vi "macro_Cmd_FindFollowHolonomicSimpleExecute.vi"() -> ()   [LabVIEW 2019, in "PathPlanner24.lvlib"]
uses:
  <vilib>/Rock Robotics/WPI/ThirdParty/JAS_Junk/TrajLib/TypeDef/CHASSIS_SPEEDS.ctl
  <vilib>/Rock Robotics/WPI/ThirdParty/JAS_Junk/TrajLib/TypeDef/POSE2D.ctl
  <vilib>/Rock Robotics/WPI/ThirdParty/JAS_Junk/TrajLib/TypeDef/TRANSLATION2D.ctl
  <vilib>/Rock Robotics/WPI/ThirdParty/JAS_Junk/TrajLib/TypeDef/ROTATION2D.ctl
  <vilib>/Rock Robotics/WPI/ThirdParty/JAS_Junk/TrajLib/ProfiledPIDController_NewPeriod.vi
  <vilib>/Rock Robotics/WPI/ThirdParty/JAS_Junk/TrajLib/ProfiledPIDController_SetIntegratorRange.vi
  <vilib>/Rock Robotics/WPI/ThirdParty/JAS_Junk/TrajLib/ProfiledPIDController_DisableContInput.vi
  <vilib>/Rock Robotics/WPI/ThirdParty/JAS_Junk/TrajLib/ProfiledPIDController_EnableContInput.vi
  <vilib>/Rock Robotics/WPI/ThirdParty/JAS_Junk/TrajLib/TrapProfConstraint_New.vi
  <vilib>/Rock Robotics/WPI/ThirdParty/JAS_Junk/TrajLib/Pose2d_New.vi
  <vilib>/Rock Robotics/WPI/ThirdParty/JAS_Junk/TrajLib/Conv_Deg_Radians.vi
  <vilib>/Rock Robotics/WPI/ThirdParty/JAS_Junk/TrajLib/TrapProfState_New.vi
  <vilib>/Rock Robotics/WPI/ThirdParty/JAS_Junk/TrajLib/PIDController_NewPeriod.vi
  <vilib>/Rock Robotics/SystemInterfaces/NetworkCommunication/NetComm_UsageReport_report.vi
  <vilib>/Rock Robotics/WPI/ThirdParty/JAS_Junk/TrajLib/PIDController_SetIntegratorRange.vi
  <vilib>/Rock Robotics/WPI/ThirdParty/JAS_Junk/TrajLib/PIDController_DisableContinousInput.vi
  <vilib>/Rock Robotics/WPI/ThirdParty/JAS_Junk/TrajLib/PIDController_EnableContinousInput.vi
  <vilib>/Rock Robotics/WPI/ThirdParty/JAS_Junk/TrajLib/Rotation2d_CreateAngle.vi
  <vilib>/Rock Robotics/WPI/ThirdParty/JAS_Junk/TrajLib/Translation2d_Create.vi
  <vilib>/Rock Robotics/WPI/ThirdParty/JAS_Junk/TrajLib/Globals/Util_LibraryGlobals.vi
  PathPlanner24.lvlib
  <vilib>/Rock Robotics/WPI/ThirdParty/JAS_Junk/TrajLib/Trajectory_Library.lvlib
panel:
  in  "Target Pose M":T1={"TRANSLATION"={"X"=0.0, "Y"=0.0}, "ROTATION"={"VALUE"=0.0, "COS"=1.0, "SIN"=0.0}} {"ROTATION"."SIN" format="%13.4f"; "ROTATION"."COS" format="%13.4f"; "ROTATION"."VALUE" format="%13.4f"; "TRANSLATION"."Y" format="%14.3f"; "TRANSLATION"."X" format="%14.3f"}
  out "Complete":bool
  in  "CurrentChassisSpeeds":T4 {"vOmega" format="%10.3f"; "vY" format="%10.3f"; "vX" format="%10.3f"}
  in  "Reset":bool
  in  "currentPose":T1={"TRANSLATION"={"X"=0.0, "Y"=0.0}, "ROTATION"={"VALUE"=0.0, "COS"=1.0, "SIN"=0.0}} {"ROTATION"."SIN" format="%13.4f"; "ROTATION"."COS" format="%13.4f"; "ROTATION"."VALUE" format="%13.4f"; "TRANSLATION"."Y" format="%14.3f"; "TRANSLATION"."X" format="%14.3f"}
  out "Position Error M":dbl
  out "At Reference":bool
  out "calcChassisSpeed":T4 {"vOmega" format="%10.3f"; "vY" format="%10.3f"; "vX" format="%10.3f"}
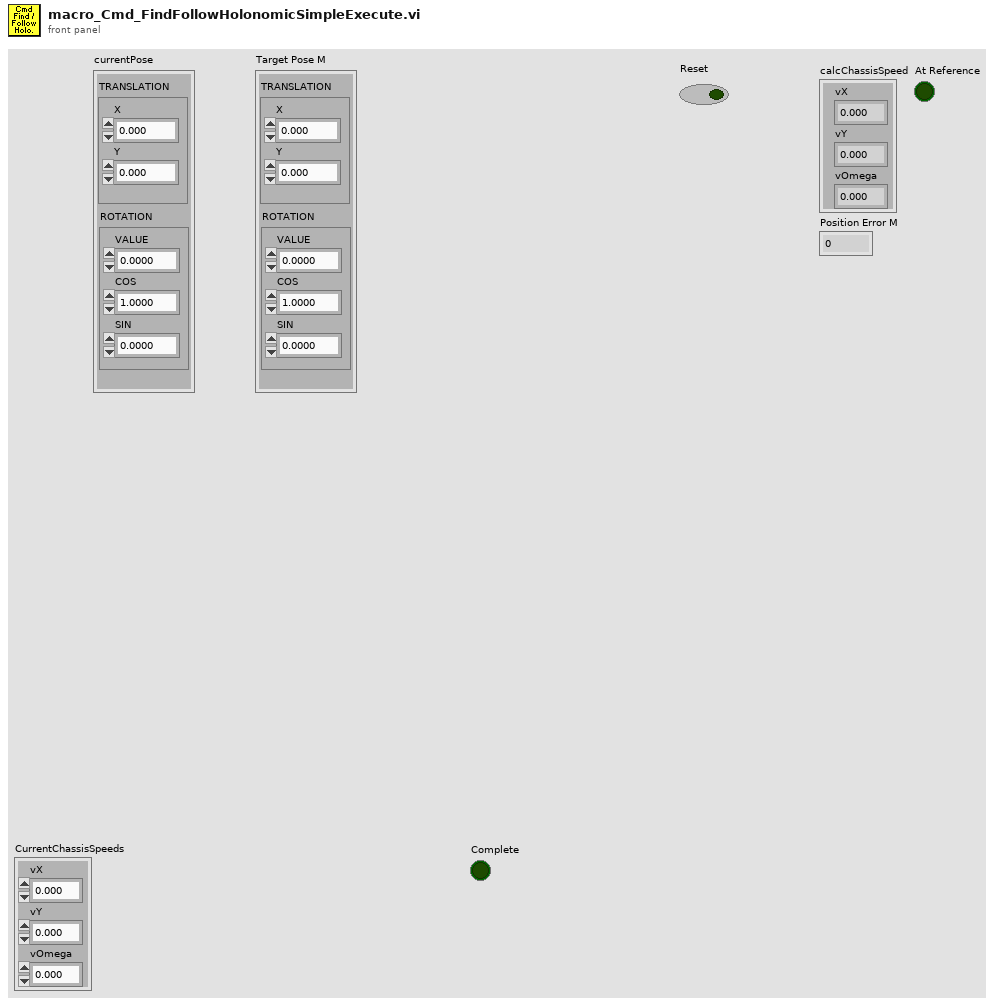
[diagram p1: front panel]
types:
  T1 = typedef "Trajectory_Library.lvlib/POSE2D.ctl" = cluster{"TRANSLATION":T2, "ROTATION":T3}
  T2 = typedef "Trajectory_Library.lvlib/TRANSLATION2D.ctl" = cluster{"X":dbl, "Y":dbl}
  T3 = typedef "Trajectory_Library.lvlib/ROTATION2D.ctl" = cluster{"VALUE":dbl, "COS":dbl, "SIN":dbl}
  T4 = typedef "Trajectory_Library.lvlib/CHASSIS_SPEEDS.ctl" = cluster{"vX":dbl, "vY":dbl, "vOmega":dbl}
  T5 = typedef "Trajectory_Library.lvlib/PID_TUNING.ctl" = cluster{"Kp":dbl, "Ki":dbl, "Kd":dbl, "MaximumIntegral":dbl, "MinimumIntegral":dbl}
  T6 = typedef "PathPlanner24.lvlib/PathPlannerReplanningConfig.ctl" = cluster{"enableInitialReplanning":bool, "enableDynamicReplanning":bool, "dynamicReplanningTotalErrorThreshold":dbl, "dynamicReplanningErrorSpikeThreshold":dbl}
  T7 = typedef "Trajectory_Library.lvlib/PROFILED_PID_CONTROLLER.ctl" = cluster{"Controller":T8, "Goal":T9, "Setpoint":T9, "Constraint":T10}
  T8 = typedef "Trajectory_Library.lvlib/PID_CONTROLLER.ctl" = cluster{"Kp":dbl, "Ki":dbl, "Kd":dbl, "Period":dbl, "Max_Integral":dbl, "Min_Integral":dbl, "Max_Input":dbl, "Min_Input":dbl, "Continuous":bool, "PositionError":dbl, "VelocityError":dbl, "PrevError":dbl, "TotalError":dbl, "PositionTolerance":dbl, "VelocityTolerance":dbl, "SetPoint":dbl, "Kf":dbl, "Prev_Deriv":dbl, "Prev_Deriv 2":dbl, "DerivativeFilter":bool, "Min_Output":dbl, "Max_Output":dbl, "Prev_F_P":dbl, "Prev_F_P_2":dbl, "AntiWindupActive":bool, "Measurement":dbl}
  T9 = typedef "Trajectory_Library.lvlib/TRAPEZOID_PROFILE_STATE.ctl" = cluster{"Position":dbl, "Velocity":dbl}
  T10 = typedef "Trajectory_Library.lvlib/TRAPEZOID_PROFILE_CONSTRAINT.ctl" = cluster{"MaxVelocity":dbl, "MaxAcceleration":dbl}
  T11 = typedef "PathPlanner24.lvlib/PathPlannerPathConstraints.ctl" = cluster{"MaxVelocityMps;":dbl, "MaxAccelerationMpsSq;":dbl, "MaxAngularVelRadPsEc;":dbl, "MaxAngularAccRadPSecSq":dbl, "Exists":bool}
  T12 = typedef "Trajectory_Library.lvlib/HOLONOMIC_PACK_TUNING.ctl" = cluster{"X PID Tuning":T5, "Y PID Tuning":T5, "thetaProfiledPID_CTRL":T7}
  T13 = typedef "PathPlanner24.lvlib/PathPlannerCmdFindConfig.ctl" = cluster{"Goal Position":T2, "GoalEndState":T14, "PathPlannerPathConstraints":T11, "Rotation Delay Distance M":dbl}
  T14 = typedef "PathPlanner24.lvlib/PathPlannerGoalEndState.ctl" = cluster{"Velocity":dbl, "Rotation":T3}
  T15 = typedef "PathPlanner24.lvlib/PathPlannerCmdFollowHolConfig.ctl" = cluster{"HOLONOMIC_CTRL_PACK_TUNING":T12, "Max Wheel Speed M/S":dbl, "Tolerance SI":T1, "Drive Base Radius M":dbl, "ControlPastEnd_Sec":dbl, "ReplanningConfig":T6, "Period_Sec":dbl, "Trigger Events":bool}
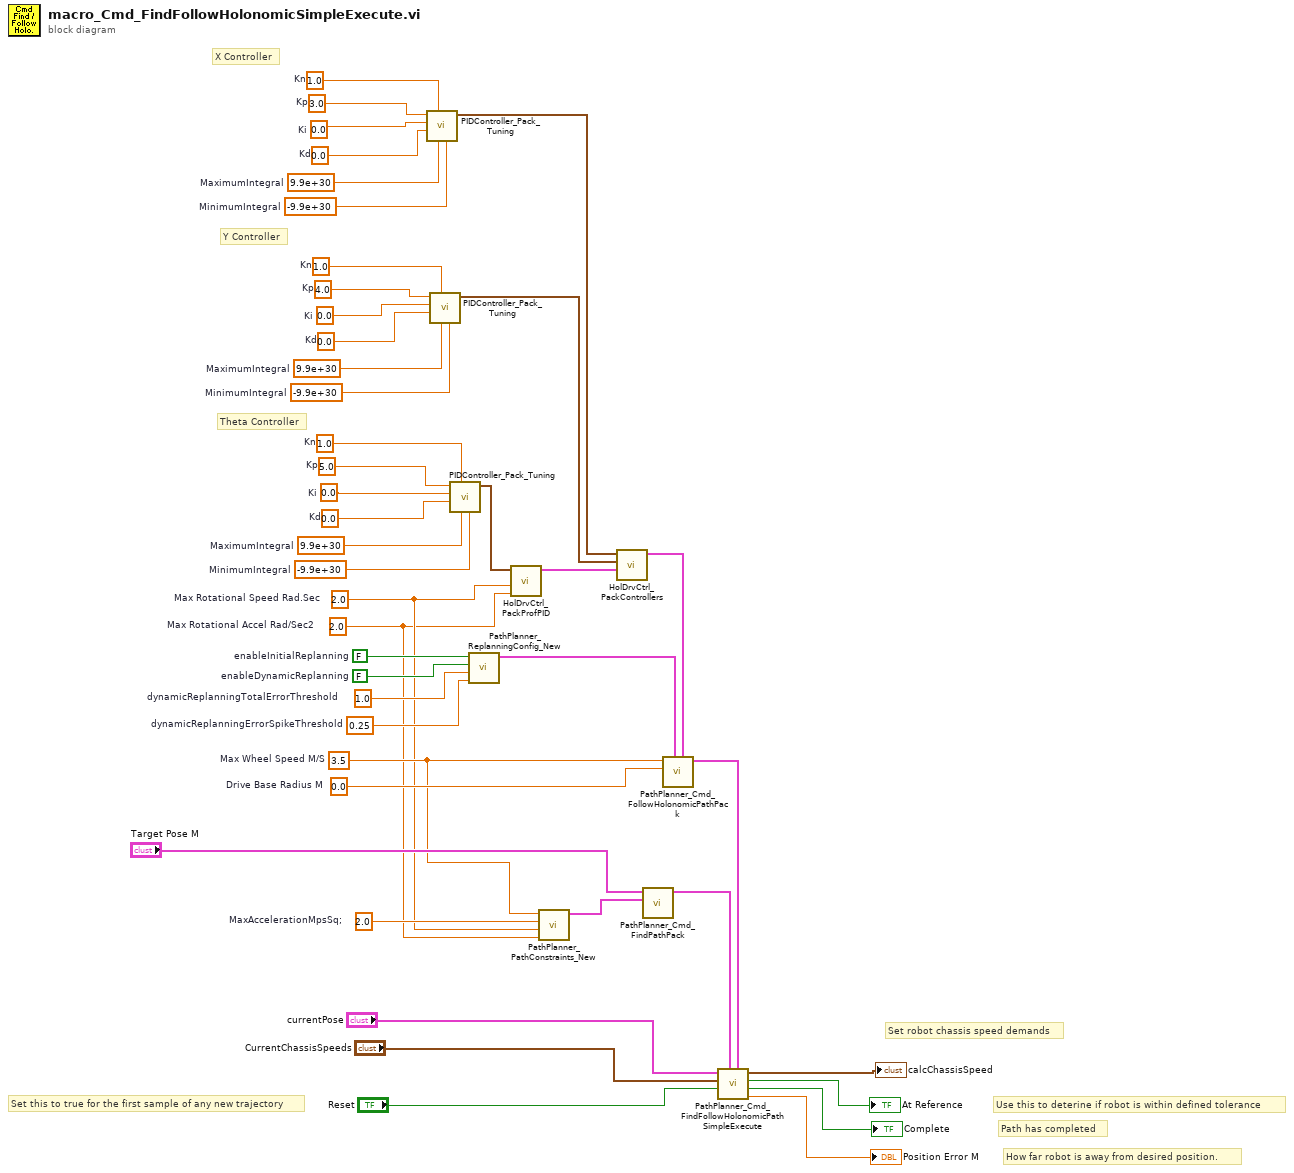
[diagram p0: block diagram]
diagram:
  w5 = 2.0  # MaxAccelerationMpsSq;
  w16 = FALSE  # enableInitialReplanning
  w17 = FALSE  # enableDynamicReplanning
  w18 = 1.0  # dynamicReplanningTotalErrorThreshold
  w19 = 0.25  # dynamicReplanningErrorSpikeThreshold
  w15 = 0.0  # Drive Base Radius M
  w3 = 3.5  # Max Wheel Speed M/S
  w29 = 1.0  # Kn
  w32 = 5.0  # Kp
  w41 = 0.0  # Ki
  w42 = 0.0  # Kd
  w43 = 9.9e+30  # MaximumIntegral
  w44 = -9.9e+30  # MinimumIntegral
  w27 = 1.0  # Kn
  w30 = 3.0  # Kp
  w33 = 0.0  # Ki
  w34 = 0.0  # Kd
  w35 = 9.9e+30  # MaximumIntegral
  w36 = -9.9e+30  # MinimumIntegral
  w28 = 1.0  # Kn
  w31 = 4.0  # Kp
  w37 = 0.0  # Ki
  w38 = 0.0  # Kd
  w39 = 9.9e+30  # MaximumIntegral
  w40 = -9.9e+30  # MinimumIntegral
  w1 = 2.0  # Max Rotational Accel Rad/Sec2
  w2 = 2.0  # Max Rotational Speed Rad.Sec
  # "Path has completed"
  # "How far robot is away from desired position."
  # "Use this to deterine if robot is within defined tolerance"
  # "Set robot chassis speed demands"
  # "Set this to true for the first sample of any new trajectory"
  # "Theta Controller"
  # "Y Controller"
  # "X Controller"
  n1 = call <vilib>:"PIDController_Pack_Tuning.vi"("MinimumIntegral"=w36, "MaximumIntegral"=w35, "Kn"=w27, "Kd"=w34, "Ki"=w33, "Kp"=w30) -> ("PID Tuning"=w23:T5)  [unwired: 5 in]
  n2 = call <vilib>:"PIDController_Pack_Tuning.vi"("MinimumIntegral"=w40, "MaximumIntegral"=w39, "Kn"=w28, "Kd"=w38, "Ki"=w37, "Kp"=w31) -> ("PID Tuning"=w22:T5)  [unwired: 5 in]
  n3 = call <vilib>:"PIDController_Pack_Tuning.vi"("MinimumIntegral"=w44, "MaximumIntegral"=w43, "Kn"=w29, "Kd"=w42, "Ki"=w41, "Kp"=w32) -> ("PID Tuning"=w26:T5)  [unwired: 5 in]
  n4 = call "PathPlanner_ReplanningConfig_New.vi"("dynamicReplanningErrorSpikeThreshold"=w19, "dynamicReplanningTotalErrorThreshold"=w18, "enableDynamicReplanning"=w17, "enableInitialReplanning"=w16) -> ("ReplanningConfig"=w20:T6)  [unwired: 7 in]
  n5 = call <vilib>:"HolDrvCtrl_PackProfPID.vi"("Max Accel"=w1, "Max Speed"=w2, "Theta PID Tuning"=w26) -> ("Theta PID CONTROLLER"=w21:T7)  [unwired: 8 in]
  n6 = call "PathPlanner_PathConstraints_New.vi"("MaxAngularAccRadPSecSq"=w1, "MaxAngularVelRadPsEc;"=w2, "MaxAccelerationMpsSq;"=w5, "MaxVelocityMps;"=w3) -> ("PathPlannerConstraints"=w4:T11)  [unwired: 7 in]
  n7 = call <vilib>:"HolDrvCtrl_PackControllers.vi"("thetaProfiledPID_CTRL"=w21, "Y PID Tuning"=w22, "X PID Tuning"=w23) -> ("HOLONOMIC_CTRL_PACK_TUNING"=w24:T12)  [unwired: 8 in]
  n8 = call "PathPlanner_Cmd_FindPathPack.vi"("PathPlannerPathConstraints"=w4, "Target Pose M"="Target Pose M") -> ("PathPlanner_Cmd_FindConfig"=w7:T13)  [unwired: 9 in]
  n9 = call "PathPlanner_Cmd_FollowHolonomicPathPack.vi"("HOLONOMIC_CTRL_PACK_TUNING"=w24, "ReplanningConfig"=w20, "Drive Base Radius M"=w15, "Max Wheel Speed M/S"=w3) -> ("PathPlanner_Ctrl_HolDrvConfig"=w25:T15)  [unwired: 7 in]
  n10 = call "PathPlanner_Cmd_FindFollowHolonomicPathSimpleExecute.vi"("PathPlanner_Cmd_FollowHolConfig"=w25, "PathPlanner_Cmd_FindConfig"=w7, "Reset"="Reset", "CurrentChassisSpeeds"="CurrentChassisSpeeds", "Current Pose SI"="currentPose") -> ("Position Error M"=→"Position Error M":dbl, "Complete"=→"Complete":bool, "At Reference"=→"At Reference":bool, "calcChassisSpeed"=→"calcChassisSpeed":T4)  [unwired: 2 in, 1 out]
